vi "recalculate.vi"() -> ()   [LabVIEW 2010]
uses:
  <vilib>/Utility/xml.llb/Read From XML File(string).vi
  <vilib>/Utility/xml.llb/Write to XML File(string).vi
  <vilib>/Analysis/NI_AALBase.lvlib
panel:
  in  "Data Flag":string(combo)
  in  "New File Directory (if saving to new file)":path caption="New File Directory"
  in  "stop":bool
  in  "Notes":string
  in  "Data File to Load":path
  out "Electrode 2 Results":T1
  out "Electrode 1 Results":T1
  in  "OK Button":bool
  in  "File Action":u16(ring) items=["None (Just Cacluate)", "New File", "Overwrite Existing File"]
  in  "Run Settings":T2={"Operator"="", "Sample (or CRM) ID"="", "Sample Temp"=0.0, "Salinity"=0.0, "Sample Units"=FALSE, "Sample Size"=0.0, "Operation Mode"=TRUE}
  in  "Configuration":T3={"Alkalinity Calculation Functions"={"HCl Temp Correction Function"="", "Sample Temp Correction Function"="", "Dosimat Correction Function"="", "Cell Temp Correction Function"="", "HCl Density Function"=""}, "Instrument Settings"={"Relay Port"="COM6", "Agilent Port"="COM5", "Dosimat Port"="COM4", "Thermal Coeffients Path"=path ""}, "Titration Settings"={"Hold Time (sec)"=300, "Initial HCl Increment"=0.0, "Target EMF"=0.0, "Agilent Monitoring Refresh Period"=0.0, "Small HCl Increment"=0.0, "Number of Titration Points"=0}, "Other Settings"={"HCl Concentration"=0.0, "HCl Lot ID"=""}, "Electrode Settings"={"Probe ID - Electrode 1 "=0, "Channel - Electrode 1"=0, "Probe ID - Electrode 2"=0, "Channel - Electrode 2"=0}} {"Electrode Settings"."Probe ID - Electrode 2" items=["OLD1", "OLD2", "OW1-10659", "OW1-10682", "OW1-10628", "OW1-10628"]; "Electrode Settings"."Probe ID - Electrode 1" items=["OLD1", "OLD2", "OW1-10659", "OW1-10682", "OW1-10628", "OW1-10628"]}
  # "Directions: \n1. First select the file that you want to recalculate from.\n2. Run the VI (arror in the top left corner of the window).\n3. Modify configuration and run setting parameters as needed.\n4. Select a file action (create new file or overwrite old file).\n5. Hit Run\n6. Get coffee...."
  # "Fill out the fields below if you are saving corrected data to a file."
  # "Add any notes about the recalculation if you are saving the file"
  # "Titration Results"
  # "End the program..."
  # "add new electrode using qc_data_accessor"
  # "This control only works when titration is not actively taking place"
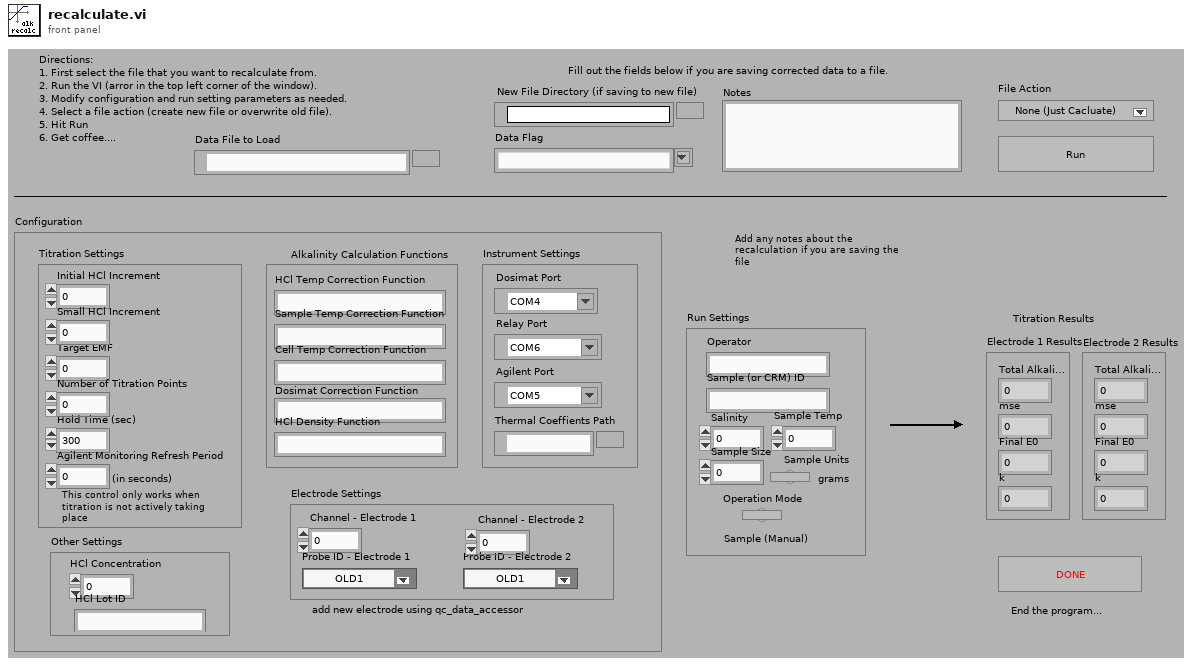
[diagram p1: front panel]
types:
  T1 = cluster{"Total Alkalinity":dbl, "mse":dbl, "Final E0":dbl, "k":dbl}
  T2 = cluster{"Operator":string, "Sample (or CRM) ID":string, "Sample Temp":dbl, "Salinity":dbl, "Sample Units":bool, "Sample Size":dbl, "Operation Mode":bool}
  T3 = cluster{"Alkalinity Calculation Functions":cluster{"HCl Temp Correction Function":string, "Sample Temp Correction Function":string, "Dosimat Correction Function":string, "Cell Temp Correction Function":string, "HCl Density Function":string}, "Instrument Settings":cluster{"Relay Port":refnum<visa-resource-name>, "Agilent Port":refnum<visa-resource-name>, "Dosimat Port":refnum<visa-resource-name>, "Thermal Coeffients Path":path}, "Titration Settings":cluster{"Hold Time (sec)":i16, "Initial HCl Increment":dbl, "Target EMF":dbl, "Agilent Monitoring Refresh Period":dbl, "Small HCl Increment":dbl, "Number of Titration Points":i32}, "Other Settings":cluster{"HCl Concentration":dbl, "HCl Lot ID":string}, "Electrode Settings":cluster{"Probe ID - Electrode 1 ":u16, "Channel - Electrode 1":i32, "Probe ID - Electrode 2":u16, "Channel - Electrode 2":i32}}
  T4 = cluster{"Run Data":cluster{"Sample (or CRM) ID":string, "Run Type (Sample or DRM)":string, "Opertator":string, "Data Flag":string, "Salinity":dbl, "Sample Temp":dbl, "Sample Size":dbl, "Sample Units":bool, "Time Completed":timestamp, "Notes":string, "Probe 1 Results":cluster{"Total Alkalinity":dbl, "mse":dbl, "Final E0":dbl, "k":dbl}, "Probe 2 Results":cluster{"Total Alkalinity":dbl, "mse":dbl, "Final E0":dbl, "k":dbl}}, "Configuration":cluster{"Alkalinity Calculation Functions":cluster{"HCl Temp Correction Function":string, "Sample Temp Correction Function":string, "Dosimat Correction Function":string, "Cell Temp Correction Function":string, "HCl Density Function":string}, "Instrument Settings":cluster{"Relay Port":refnum<visa-resource-name>, "Agilent Port":refnum<visa-resource-name>, "Dosimat Port":refnum<visa-resource-name>, "Thermal Coeffients Path":path}, "Titration Settings":cluster{"Hold Time (sec)":i16, "Initial HCl Increment":dbl, "Target EMF":dbl, "Agilent Monitoring Refresh Period":dbl, "Small HCl Increment":dbl, "Number of Titration Points":i32}, "Other Settings":cluster{"HCl Concentration":dbl, "HCl Lot ID":string}, "Electrode Settings":cluster{"Probe ID - Electrode 1 ":u16, "Channel - Electrode 1":i32, "Probe ID - Electrode 2":u16, "Channel - Electrode 2":i32}}, "Agilent Monitoring Record":cluster{"Time Stamp":timestamp, "Titration Stage":string, "Average Voltage":dbl, "Burette Temp Average":dbl, "Voltage 1":dbl, "Voltage 2":dbl, "Voltage 1 StandDev":dbl, "Voltage 2 StandDev":dbl, "Burette Temp 1":dbl, "Burette Temp 2":dbl, "Cell Temp":dbl, "Acid Temp":dbl, "Room Temp":dbl}[], "Titration Points":cluster{"Cell Temps":dbl[], "Total HCl Volumes (uncorr)":dbl[], "EMF Array 1":dbl[], "EMF Array 2":dbl[]}, string}
  T5 = cluster{"Sample (or CRM) ID":string, "Run Type (Sample or DRM)":string, "Opertator":string, "Data Flag":string, "Salinity":dbl, "Sample Temp":dbl, "Sample Size":dbl, "Sample Units":bool, "Time Completed":timestamp, "Notes":string, "Probe 1 Results":cluster{"Total Alkalinity":dbl, "mse":dbl, "Final E0":dbl, "k":dbl}, "Probe 2 Results":cluster{"Total Alkalinity":dbl, "mse":dbl, "Final E0":dbl, "k":dbl}}
  T6 = cluster{"Time Stamp":timestamp, "Titration Stage":string, "Average Voltage":dbl, "Burette Temp Average":dbl, "Voltage 1":dbl, "Voltage 2":dbl, "Voltage 1 StandDev":dbl, "Voltage 2 StandDev":dbl, "Burette Temp 1":dbl, "Burette Temp 2":dbl, "Cell Temp":dbl, "Acid Temp":dbl, "Room Temp":dbl}[]
  T7 = cluster{"Cell Temps":dbl[], "Total HCl Volumes (uncorr)":dbl[], "EMF Array 1":dbl[], "EMF Array 2":dbl[]}
  T8 = cluster{"HCl Temp Correction Function":string, "Sample Temp Correction Function":string, "Dosimat Correction Function":string, "Cell Temp Correction Function":string, "HCl Density Function":string}
  T9 = cluster{"HCl Concentration":dbl, "HCl Lot ID":string}
  T10 = cluster{"Time Stamp":timestamp, "Titration Stage":string, "Average Voltage":dbl, "Burette Temp Average":dbl, "Voltage 1":dbl, "Voltage 2":dbl, "Voltage 1 StandDev":dbl, "Voltage 2 StandDev":dbl, "Burette Temp 1":dbl, "Burette Temp 2":dbl, "Cell Temp":dbl, "Acid Temp":dbl, "Room Temp":dbl}
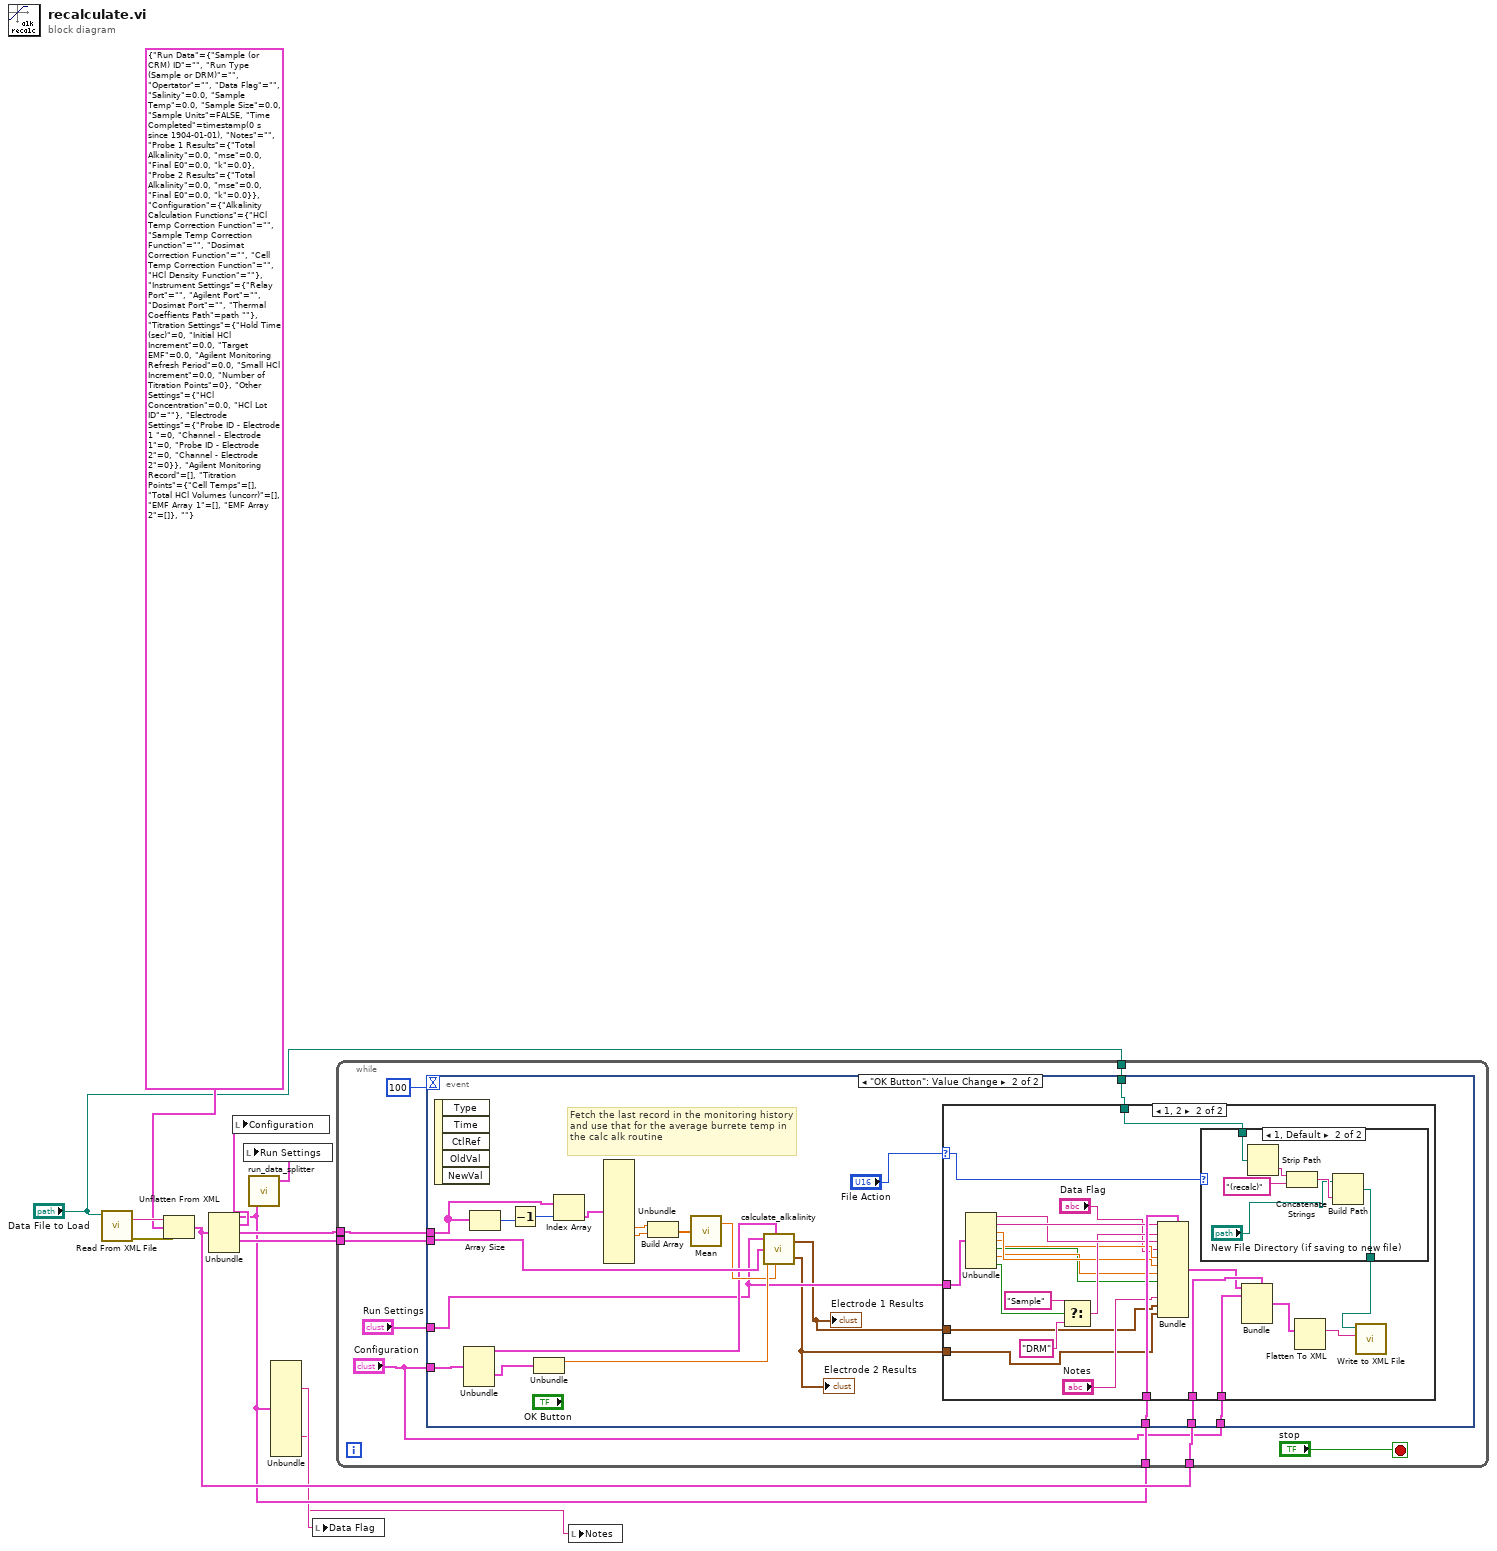
[diagram p0: block diagram]
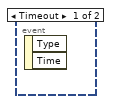
[diagram p2: hidden frame]
diagram:
  n1 = call-poly <vilib>:"Read From XML File.vi"("XML File Path"="Data File to Load") -> ("error out"=w12:errorcluster, "XML Elements"=w11:string)  [unwired: 8 in, 1 out]
  n2 = Unflatten From XML(xml string=w11, type=T4 {"Run Data"={"Sample (or CRM) ID"="", "Run Type (Sample or DRM)"="", "Opertator"="", "Data Flag"="", "Salinity"=0.0, "Sample Temp"=0.0, "Sample Size"=0.0, "Sample Units"=FALSE, "Time Completed"=timestamp(0 s since 1904-01-01), "Notes"="", "Probe 1 Results"={"Total Alkalinity"=0.0, "mse"=0.0, "Final E0"=0.0, "k"=0.0}, "Probe 2 Results"={"Total Alkalinity"=0.0, "mse"=0.0, "Final E0"=0.0, "k"=0.0}}, "Configuration"={"Alkalinity Calculation Functions"={"HCl Temp Correction Function"="", "Sample Temp Correction Function"="", "Dosimat Correction Function"="", "Cell Temp Correction Function"="", "HCl Density Function"=""}, "Instrument Settings"={"Relay Port"="", "Agilent Port"="", "Dosimat Port"="", "Thermal Coeffients Path"=path ""}, "Titration Settings"={"Hold Time (sec)"=0, "Initial HCl Increment"=0.0, "Target EMF"=0.0, "Agilent Monitoring Refresh Period"=0.0, "Small HCl Increment"=0.0, "Number of Titration Points"=0}, "Other Settings"={"HCl Concentration"=0.0, "HCl Lot ID"=""}, "Electrode Settings"={"Probe ID - Electrode 1 "=0, "Channel - Electrode 1"=0, "Probe ID - Electrode 2"=0, "Channel - Electrode 2"=0}}, "Agilent Monitoring Record"=[], "Titration Points"={"Cell Temps"=[], "Total HCl Volumes (uncorr)"=[], "EMF Array 1"=[], "EMF Array 2"=[]}, ""} ("output cluster"), error in (no error)=w12) -> (value=w5:T4)  [unwired: 1 out]
  n3 = Unbundle(w5) -> ("Run Data"=w3:T5, "Configuration"=w9:T3, "Agilent Monitoring Record"=w6:T6, "Titration Points"=w7:T7)  [unwired: 1 out]
  n4 = local write "Configuration"(w9) -> ()
  n5 = call "run_data_splitter.vi"("Run Data"=w3) -> ("Run Settings"=w8:T2)  [unwired: 2 in]
  n6 = local write "Run Settings"(w8) -> ()
  n7 = Unbundle(w3) -> ("Data Flag"=w2:string, "Notes"=w1:string)  [unwired: 10 out]
  n8 = local write "Data Flag"(w2) -> ()
  n9 = while {
    tunnel: w7 -> [w19]
    tunnel: w6 -> [w18]
    tunnel: w5 -> [w17]
    tunnel: w3 -> [w16]
    tunnel: "Data File to Load" -> [w13]
    stop <- "stop" stop-if-true
    n10 = event shown="[1] \"OK Button\": Value Change" {
      selector: _ -> [_ _]
      dyn-events: _ -> [_ _]
      timeout: 100 -> [_ _]
      tunnel: "Run Settings" -> [_ w27]
      tunnel: w19 -> [_ w42]
      tunnel: w18 -> [_ w38]
      tunnel: "Configuration" -> [_ w32]
      tunnel: w17 -> [_ w29]
      tunnel: w16 -> [_ w28]
      tunnel: "Configuration" -> [_ w24]
      tunnel: w13 -> [_ w22]
      event Timeout {
        n11 = event-data() -> ()  [unwired: 1 in, 2 out]
      }
      event "OK Button": Value Change {
        # "Fetch the last record in the monitoring history and use that for the average burrete temp in the calc alk routine"
        n12 = event-data() -> ()  [unwired: 1 in, 5 out]
        n13 = Unbundle(w32) -> ("Alkalinity Calculation Functions"=w31:T8, "Other Settings"=w30:T9)  [unwired: 3 out]
        n14 = Array Size(array=w38) -> (size(s)=w40:i32)
        n15 = Decrement(x=w40) -> (x-1=w39:i32)
        n16 = Unbundle(w30) -> ("HCl Concentration"=w41:dbl)  [unwired: 1 out]
        n17 = Index Array(array=w38, index=w39) -> (element=w37:T10)
        n18 = Unbundle(w37) -> ("Burette Temp 1"=w36:dbl, "Burette Temp 2"=w35:dbl)  [unwired: 11 out]
        n19 = Build Array(w36, w35) -> (w34:dbl[])
        n20 = call <vilib>:"Mean.vi"("X"=w34) -> ("mean"=w33:dbl)  [unwired: 1 out]
        n21 = call "calculate_alkalinity.vi"("Run Settings"=w27, "Alkalinity Calculation Functions"=w31, "Titration Points"=w42, "HCl Concentration"=w41, "HCl Temp (uncorr)"=w33) -> ("Probe 1 Results"=w26:T1, "Probe 2 Results"=w25:T1)
        "Electrode 1 Results" <- w26
        "Electrode 2 Results" <- w25
        n22 = case shown="1, 2" "File Action" {
          selector: "File Action" -> [_ w46]
          tunnel: w29 -> [_ w64]
          tunnel: w28 -> [_ w62]
          tunnel: w27 -> [_ w61]
          tunnel: w26 -> [_ w49]
          tunnel: w25 -> [_ w48]
          tunnel: w24 -> [_ w47]
          tunnel: w22 -> [_ w45]
          frame 0, Default {
          }
          frame 1, 2 {
            n23 = Unbundle(w61) -> ("Operator"=w59:string, "Sample (or CRM) ID"=w60:string, "Sample Temp"=w54:dbl, "Salinity"=w53:dbl, "Sample Units"=w51:bool, "Sample Size"=w52:dbl, "Operation Mode"=w56:bool)
            n24 = Select(t="Sample", s=w56, f="DRM") -> (s? t:f=w55:string)
            n25 = Bundle(cluster=w62, "Sample (or CRM) ID"=w60, "Run Type (Sample or DRM)"=w55, "Opertator"=w59, "Data Flag"="Data Flag", "Salinity"=w53, "Sample Temp"=w54, "Sample Size"=w52, "Sample Units"=w51, "Notes"="Notes", "Probe 1 Results"=w49, "Probe 2 Results"=w48) -> (w63:T5)  [unwired: 1 in]
            n26 = case shown="1, Default" w46 {
              tunnel: w45 -> [w67 w73]
              tunnel: [w67 w69] -> w44
              frame 2 {
              }
              frame 1, Default {
                n27 = Strip Path(path=w73) -> (name=w72:string)  [unwired: 1 out]
                n28 = Concatenate Strings(w72, "(recalc)") -> (w70:string)
                n29 = Build Path(base path="New File Directory (if saving to new file)", name or relative path=w70) -> (appended path=w69:path)
              }
            }
            n30 = Bundle(cluster=w64, "Run Data"=w63, "Configuration"=w47) -> (w66:T4)  [unwired: 3 in]
            n31 = Flatten To XML(anything=w66) -> (xml string=w65:string)
            n32 = call-poly <vilib>:"Write to XML File.vi"("XML Input"=w65, "XML File Path"=w44) -> ()  [unwired: 7 in, 3 out]
          }
        }
      }
    }
  }
  n33 = local write "Notes"(w1) -> ()
